vi "Read XML_Extra Checks_Check Parameter Name Uniqueness_create SDI string.vi"(9 "SDIValue":u8, 11 "SDI_Enabled":bool) -> (3 "SDI String":string)   [LabVIEW 2016]
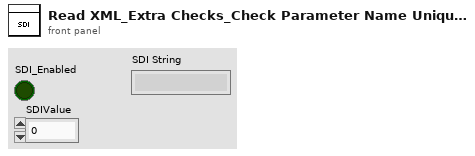
[diagram p1: front panel]
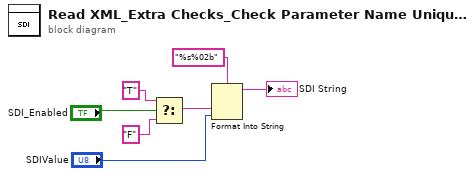
[diagram p0: block diagram]
diagram:
  n1 = Select(t="T", s="SDI_Enabled", f="F") -> (s? t:f=w4:string)
  n2 = Format Into String(format string="%s%02b", w4, "SDIValue") -> (resulting string=→"SDI String":string)  [unwired: 2 in, 1 out]
